vi "Get Return - Integer.vi"(7 "Function Name":string, 8 "Error In":errorcluster, 11 "OPI Ref":refnum<data-value>) -> (0 "Error Out":errorcluster, 1 "Return Value":i64 caption="Integer", 3 "OPI Ref":refnum<data-value>)   [LabVIEW 2012, in "OPI.lvclass"]
doc: "Get return value from previously made function call, specified by Function Name. \n\nReturn an integer - LabVIEW I64 representation."
uses:
  OPI.lvclass
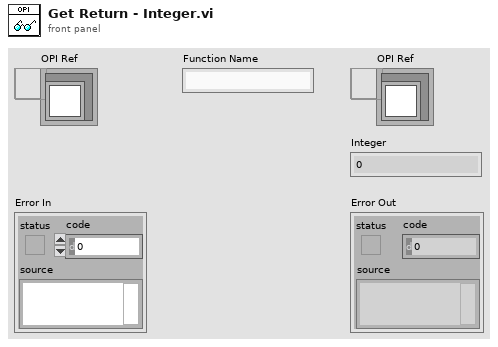
[diagram p1: front panel]
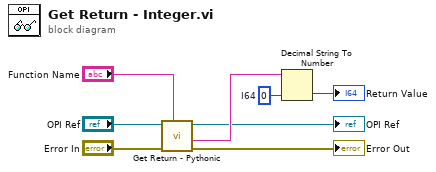
[diagram p0: block diagram]
diagram:
  w4 = i64 0  # I64
  n1 = call "Get Return - Pythonic.vi"("Function Name"="Function Name", "Error In"="Error In", "OPI Ref"="OPI Ref") -> ("Error Out"=→"Error Out":errorcluster, "Pythonic Return Value"=w5:string, "OPI Ref"=→"OPI Ref":refnum<data-value>)  [unwired: 6 in]
  n2 = Decimal String To Number(string=w5, default (0L)=w4) -> (number=→"Return Value":i64)  [unwired: 1 in, 1 out]
